vi "tool_Unicode_Convert Unicode to ASCII (1D).vi"(4 "Unicode":string[](array[string])) -> (1 "ASCII":string[](array[string]))   [LabVIEW 2020]
uses:
  kernel32.dll
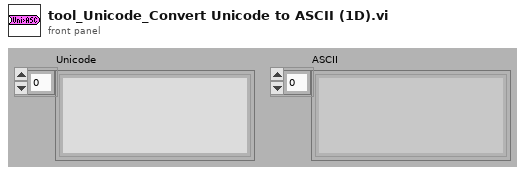
[diagram p1: front panel]
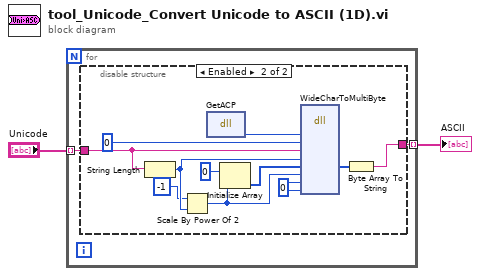
[diagram p0: block diagram]
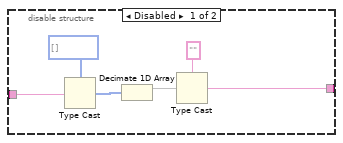
[diagram p2: hidden frame]
diagram:
  n1 = for {
    tunnel: "Unicode" -> [w4] mode=indexing
    tunnel: [w3] -> w1 mode=indexing
    n2 = disable-structure shown="Enabled" {
      disable-tunnel: w4 -> [w10 w16]
      disable-tunnel: [w7 w15] -> w3
      frame Disabled {
        n3 = Type Cast(type=u8[] [], x=w10) -> (*(type *) &x=w6:u8[])
        n4 = Decimate 1D Array(w6) -> (w5:u8[])  [unwired: 1 out]
        n5 = Type Cast(type="", x=w5) -> (*(type *) &x=w7:string)
      }
      frame Enabled {
        w11 = u32 0
        n6 = String Length(string=w16) -> (length=w14:i32)
        n7 = Scale By Power Of 2(n=-1, x=w14) -> (x*2^n=w12:i32)
        n8 = dll-call lib="kernel32.dll" fn="GetACP" label="GetACP()"() -> (w21:u32)  [unwired: 3 in, 2 out]
        n9 = Initialize Array(u8 0, w12) -> (w19:u8[])
        n10 = dll-call lib="kernel32.dll" fn="WideCharToMultiByte"("codePage"=w21, "dwFlags"=u32 0, "lpWideCharStr"=w16, "cchWideChar"=w14, "lpMultiByteStr"=w19, "cbMultiByte"=w12, "lpDefaultChar"=w11, "lpUsedDefaultChar"=w11) -> ("lpMultiByteStr"=w20:u8[])  [unwired: 10 in, 3 out]
        n11 = Byte Array To String(unsigned byte array=w20) -> (string=w15:string)
      }
    }
  }
  "ASCII" <- w1
